vi "Report.vi"(8 "error in":errorcluster, 9 "Received":path, 10 "Approved":path, 11 "Report With LVCompare in":refnum<class "Report With LVCompare.lvclass">) -> (0 "error out":errorcluster, 2 "Worked?":bool, 3 "Report With LVCompare out":refnum<class "Report With LVCompare.lvclass">)   [LabVIEW 2020, in "Approval Tests.lvlib" / "Report With LVCompare.lvclass"]
uses:
  Report With LVCompare.lvclass
panel:
  out "standard error":string
  out "standard output":string
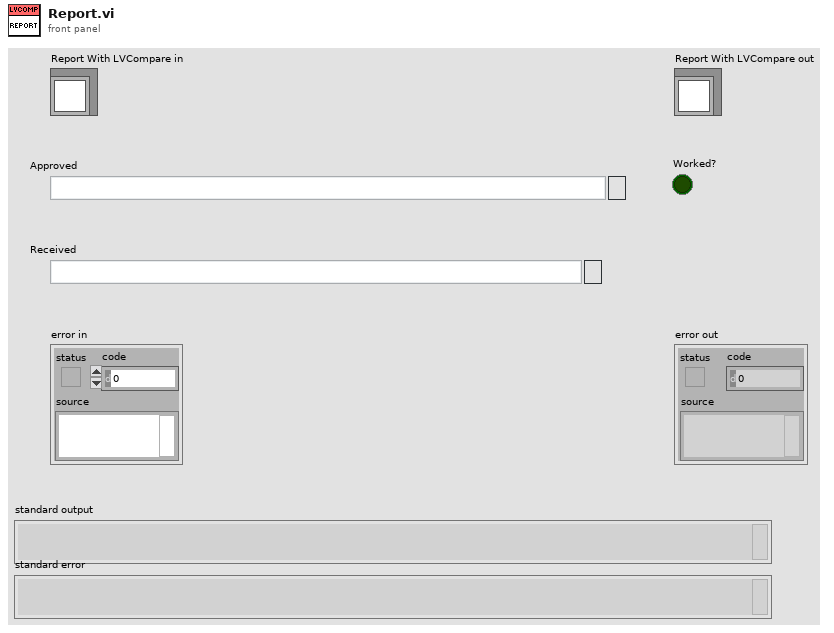
[diagram p1: front panel]
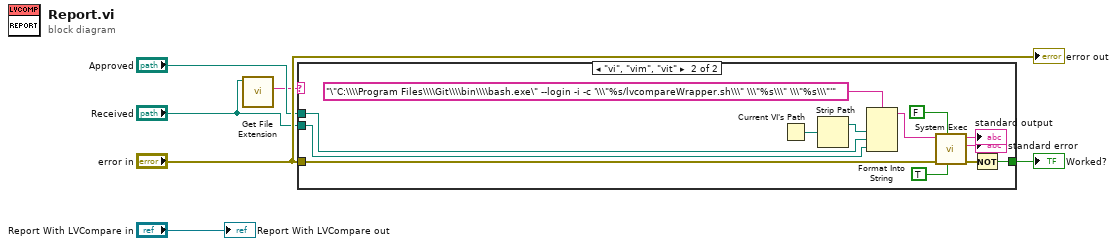
[diagram p0: block diagram]
diagram:
  n1 = call <vilib>:"Get File Extension.vi"("file"="Received") -> ("lowercase file extension"=w1:string)  [unwired: 6 in, 4 out]
  n2 = case shown="\"vi\", \"vim\", \"vit\"" w1 {
    tunnel: [_ w12] -> w4
    tunnel: "error in" -> [_ w18]
    tunnel: "Approved" -> [_ w11]
    tunnel: "Received" -> [_ w10]
    frame Default {
    }
    frame "vi", "vim", "vit" {
      n3 = Current VI's Path() -> (path=w15:path)
      n4 = Strip Path(path=w15) -> (stripped path=w14:path)  [unwired: 1 out]
      n5 = Format Into String(format string="\"C:\\\\Program Files\\\\Git\\\\bin\\\\bash.exe\" --login -i -c '\\\"%s/lvcompareWrapper.sh\\\" \\\"%s\\\" \\\"%s\\\"'", w14, w11, w10) -> (resulting string=w16:string)  [unwired: 2 in, 1 out]
      n6 = call <vilib>:"System Exec.vi"("run minimized? (F)"=TRUE, "wait until completion? (T)"=FALSE, "error in (no error)"=w18, "command line"=w16) -> ("error out"=w19:errorcluster, "standard error"=→"standard error":string, "standard output"=→"standard output":string)  [unwired: 4 in, 1 out]
      n7 = Not(x=w19) -> (.not. x?=w12:bool)
    }
  }
  "Worked?" <- w4
  "error out" <- "error in"
  "Report With LVCompare out" <- "Report With LVCompare in"
